vi "Register gRPC Methods.vi"(8 "error in (no error)":errorcluster, 11 "Template Server in":refnum<class "Template Server.lvclass">) -> (0 "error out":errorcluster, 3 "Template Server out":refnum<class "Template Server.lvclass">)   [LabVIEW 2019, in "Template Server.lvlib" / "Template Server.lvclass"]
uses:
  Template Server.lvclass
  typeDefs/Server Internal Message.ctl
  typeDefs/Server Internal Message UE.ctl
  typeDefs/Server Internal UEs.ctl
  <vilib>/gRPC/LabVIEW gRPC Library/Shared/grpcId.ctl
  <vilib>/gRPC/LabVIEW gRPC Library/grpc-lvsupport-release.lvlib
  <vilib>/gRPC/LabVIEW gRPC Library/Server API/typeDefs/gRPCId Cluster.ctl
  <vilib>/gRPC/LabVIEW gRPC Library/Server API/typeDefs/gRPCId Cluster UE.ctl
  typeDefs/Server gRPC UEs.ctl
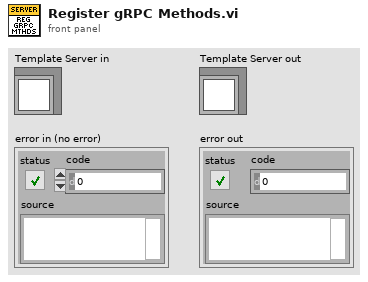
[diagram p1: front panel]
types:
  T1 = typedef "Template Server.lvlib/Template Server.lvclass/Server gRPC UEs.ctl" = cluster{"Template gRPCId UE":T2}
  T2 = typedef "grpc-lvsupport-release.lvlib/gRPCId Cluster UE.ctl" = refnum<user-event>
  T3 = typedef "Template Server.lvlib/Template Server.lvclass/Server Internal UEs.ctl" = cluster{"Template Internal UE":T4}
  T4 = typedef "Template Server.lvlib/Template Server.lvclass/Server Internal Message UE.ctl" = refnum<user-event>
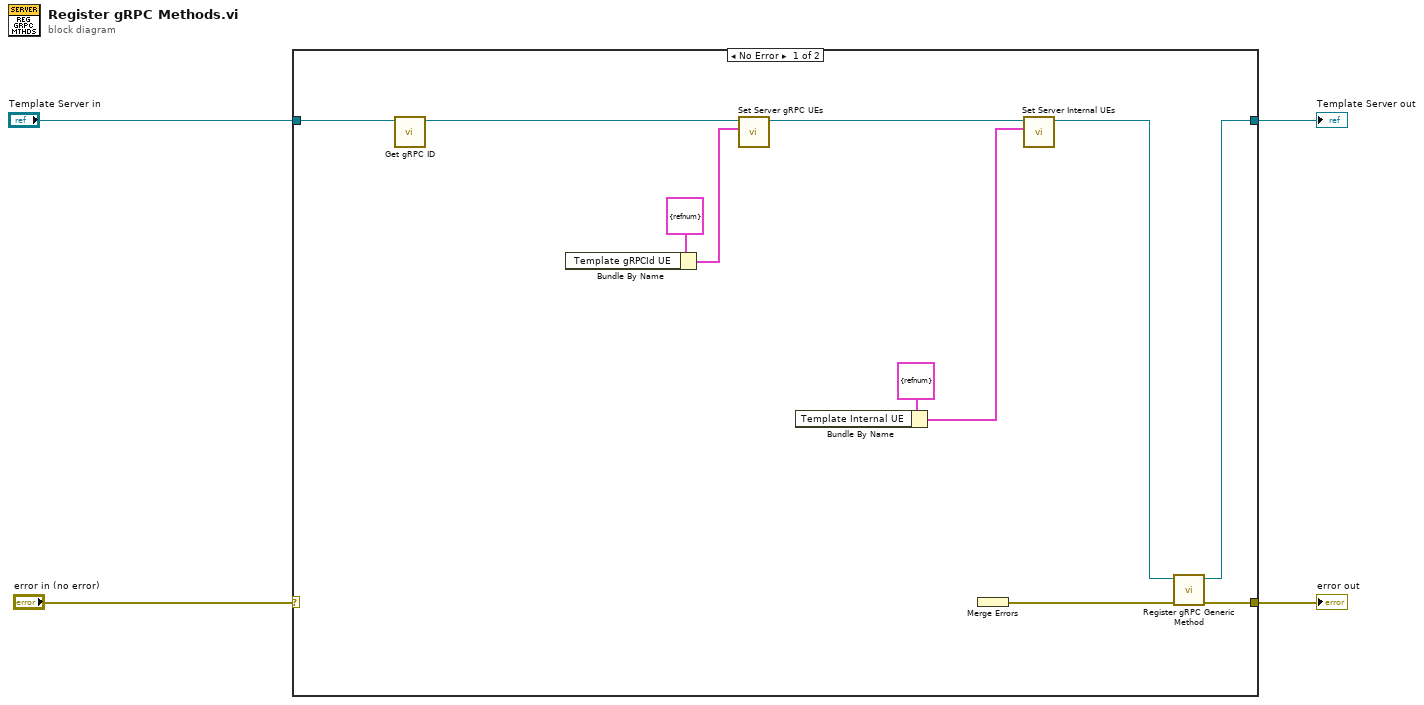
[diagram p0: block diagram]
diagram:
  n1 = case shown="No Error" "error in (no error)" {
    selector: "error in (no error)" -> [_ w16]
    tunnel: "Template Server in" -> [w14 w17]
    tunnel: [w7 w16] -> w3
    tunnel: [w5 w17] -> w2
    frame No Error {
      n2 = call "Get gRPC ID.vi"("OOP Server in"=w14) -> ("OOP Server out"=w15:refnum<class "Template Server.lvclass">)  [unwired: 9 in, 1 out]
      n3 = Bundle By Name ("Bundle gRPC UEs")(cluster=T1 {"Template gRPCId UE"=refnum} ("gRPC Server Method Events")) -> (w10:T1)  [unwired: 1 in]
      n4 = call "Set Server gRPC UEs.vi"("Server RPC Methods"=w10, "OOP Server in"=w15) -> ("OOP Server out"=w11:refnum<class "Template Server.lvclass">)  [unwired: 9 in]
      n5 = Bundle By Name ("Bundle Internal UEs")(cluster=T3 {"Template Internal UE"=refnum} ("Server Internal UEs")) -> (w13:T3)  [unwired: 1 in]
      n6 = Merge Errors() -> (w8:errorcluster)  [unwired: 1 in]
      n7 = call "Set Server Internal UEs.vi"("Server Internal UEs"=w13, "OOP Server in"=w11) -> ("OOP Server out"=w6:refnum<class "Template Server.lvclass">)  [unwired: 9 in]
      n8 = call "Register gRPC Generic Method.vi"("error in (no error)"=w8, "Template Server in"=w6) -> ("error out"=w7:errorcluster, "Template Server out"=w5:refnum<class "Template Server.lvclass">)  [unwired: 8 in]
    }
    frame Error {
    }
  }
  "error out" <- w3
  "Template Server out" <- w2
